vi "create_Karte.vi"() -> ()   [LabVIEW 2019]
uses:
  Karte.ctl
  Kreuzung.ctl
  Koordinate.ctl
  Strasse.ctl
  Verbindung.ctl
  Strassentyp.ctl
  Haus.ctl
  <vilib>/Utility/file.llb/Read Delimited Spreadsheet (string).vi
  <vilib>/Utility/xml.llb/Write to XML File(string).vi
panel:
  out "error out":errorcluster
  in  "OK Button":bool
  in  "Table Control":string[][](table)=[["", "", "", "", "", "", "", "s", "", "", "", "", "", "", "", "", "", "", "", "", "", "", "", "", ""], ["", "", "i", "", "", "", "", "", "", "", "", "", "", "", "", "", "", "", "", "", "", "", "", "", ""], ["", "i", "", "i", "", "", "", "", "", "", "i", "", "", "", "", "", "", "", "", "", "", "", "", "", ""], ["", "", "i", "", "i", "", "", "", "", "", "", "", "", "", "", "", "", "", "", "", "", "", "", "", ""], ["", "", "", "i", "", "", "", "", "", "", "", "", "", "", "", "", "", "", "", "", "", "", "", "", ""], ["", "", "", "", "", "", "s", "", "", "", "", "", "", "", "", "", "", "", "", "", "", "", "", "", ""], ["", "", "", "", "", "s", "", "s", "s", "", "", "", "", "", "", "", "", "", "", "", "", "", "", "", ""], ["s", "", "", "", "", "", "s", "", "", "", "", "", "", "", "", "", "", "", "", "", "", "", "", "", ""], ["", "", "", "", "", "", "s", "", "", "i", "", "", "", "", "", "", "", "", "s", "", "", "", "", "", ""], ["", "", "", "", "", "", "", "", "i", "", "i", "i", "", "", "", "", "", "", "", "", "", "", "", "", ""], ["", "", "i", "", "", "", "", "", "", "i", "", "", "i", "", "", "", "", "", "", "", "", "", "", "", ""], ["", "", "", "", "", "", "", "", "", "i", "", "", "i", "", "", "", "", "i", "", "", "", "", "", "", ""], ["", "", "", "", "", "", "", "", "", "", "i", "i", "", "i", "", "", "", "", "", "", "", "", "", "", ""], ["", "", "", "", "", "", "", "", "", "", "", "", "i", "", "i", "i", "", "", "", "", "", "", "", "", ""], ["", "", "", "i", "", "", "", "", "", "", "", "", "", "i", "", "", "", "", "", "", "", "", "", "", ""], ["", "", "", "", "", "", "", "", "", "", "", "", "", "i", "", "", "s", "", "", "", "", "", "", "s", ""], ["", "", "", "", "", "", "", "", "", "", "", "", "", "", "", "s", "", "", "", "", "", "", "", "", ""], ["", "", "", "", "", "", "", "", "", "", "", "i", "", "", "", "", "", "", "", "", "", "", "", "", ""], ["", "", "", "", "", "", "", "", "s", "", "", "", "", "", "", "", "", "", "", "", "", "", "", "", ""], ["", "", "", "", "", "", "", "", "", "", "", "", "", "", "", "", "", "", "", "", "a", "a", "", "", ""], ["", "", "", "", "", "", "", "", "", "", "", "", "", "", "", "", "", "", "", "a", "", "", "a", "", ""], ["", "", "", "", "", "", "", "", "", "", "", "", "", "", "", "", "", "", "", "a", "", "", "", "", ""], ["", "", "", "", "", "", "", "", "", "", "", "", "", "", "", "", "", "", "", "", "a", "", "", "a", ""], ["", "", "", "", "", "", "", "", "", "", "", "", "", "", "", "s", "", "", "", "", "", "", "a", "", "a"], ["", "", "", "", "", "", "", "", "", "", "", "", "", "", "", "", "", "", "", "", "", "", "", "a", ""]]
  in  "Nr Häuser":i32=20
  in  "Nr Kreuzungen":i32=25
  out "all rows":string[][](array[string])=[["Nr.", "X-DIM", "Y-DIM", "Typ", "", "", ""], ["A1", "100", "40", "Strasse", "", "", ""], ["A2", "180", "70", "Strasse", "", "", ""], ["A3", "210", "70", "Strasse", "", "", ""], ["A4", "300", "70", "Strasse", "", "", ""], ["A5", "320", "70", "Strasse", "", "", ""], ["A6", "40", "100", "Strasse", "", "", ""], ["A7", "90", "100", "Strasse", "", "", ""], ["A8", "100", "100", "Strasse", "", "", ""], ["A9", "90", "170", "Strasse", "", "", ""], ["A10", "180", "170", "Strasse", "", "", ""], ["A11", "210", "170", "Strasse", "", "", ""], ["A12", "180", "190", "Strasse", "", "", ""], ["A13", "210", "190", "Strasse", "", "", ""], ["A14", "270", "190", "Strasse", "", "", ""], ["A15", "300", "190", "Strasse", "", "", ""], ["A16", "270", "230", "Strasse", "", "", ""], ["A17", "340", "230", "Strasse", "", "", ""], ["A18", "180", "240", "Strasse", "", "", ""], ["A19", "90", "260", "Strasse", "", "", ""], ["A20", "60", "320", "Strasse", "", "", ""], ["A21", "160", "320", "Strasse", "", "", ""], ["A22", "60", "360", "Strasse", "", "", ""], ["A23", "160", "400", "Strasse", "", "", ""], ["A24", "270", "400", "Strasse", "", "", ""], ["A25", "340", "400", "Strasse", "", "", ""], ["B1", "160", "0", "Haus", "", "", ""], ["B2", "220", "0", "Haus", "", "", ""], ["B3", "220", "0", "Haus", "", "", ""], ["B4", "280", "0", "Haus", "", "", ""], ["B5", "280", "0", "Haus", "", "", ""], ["B6", "340", "0", "Haus", "", "", ""], ["B7", "20", "20", "Haus", "", "", ""], ["B8", "80", "20", "Haus", "", "", ""], ["B9", "190", "20", "Haus", "", "", ""], ["B10", "250", "20", "Haus", "", "", ""], ["B11", "310", "20", "Haus", "", "", ""], ["B12", "220", "40", "Haus", "", "", ""], ["B13", "280", "40", "Haus", "", "", ""], ["B14", "50", "40", "Haus", "", "", ""], ["B15", "120", "40", "Haus", "", "", ""], ["B16", "160", "40", "Haus", "", "", ""], ["B17", "220", "40", "Haus", "", "", ""], ["B18", "280", "40", "Haus", "", "", ""], ["B19", "340", "40", "Haus", "", "", ""], ["B20", "340", "40", "Haus", "", "", ""], ["B21", "160", "40", "Haus", "", "", ""], ["B22", "380", "40", "Haus", "", "", ""], ["B23", "20", "60", "Haus", "", "", ""], ["B24", "80", "60", "Haus", "", "", ""], ["B25", "140", "70", "Haus", "", "", ""], ["B26", "360", "70", "Haus", "", "", ""], ["B27", "160", "100", "Haus", "", "", ""], ["B28", "380", "100", "Haus", "", "", ""], ["B29", "120", "100", "Haus", "", "", ""], ["B30", "120", "100", "Haus", "", "", ""], ["B31", "180", "100", "Haus", "", "", ""], ["B32", "240", "100", "Haus", "", "", ""], ["B33", "340", "100", "Haus", "", "", ""], ["B34", "380", "100", "Haus", "", "", ""], ["B35", "280", "100", "Haus", "", "", ""], ["B36", "320", "100", "Haus", "", "", ""], ["B37", "20", "120", "Haus", "", "", ""], ["B38", "60", "120", "Haus", "", "", ""], ["B39", "150", "120", "Haus", "", "", ""], ["B40", "350", "120", "Haus", "", "", ""], ["B41", "260", "130", "Haus", "", "", ""], ["B42", "180", "140", "Haus", "", "", ""], ["B43", "120", "140", "Haus", "", "", ""], ["B44", "320", "140", "Haus", "", "", ""], ["B45", "320", "140", "Haus", "", "", ""], ["B46", "380", "140", "Haus", "", "", ""], ["B47", "360", "140", "Haus", "", "", ""], ["B48", "40", "150", "Haus", "", "", ""], ["B49", "280", "160", "Haus", "", "", ""], ["B50", "240", "160", "Haus", "", "", ""], ["B51", "340", "170", "Haus", "", "", ""], ["B52", "20", "180", "Haus", "", "", ""], ["B53", "60", "180", "Haus", "", "", ""], ["B54", "45", "180", "Haus", "", "", ""], ["B55", "5", "180", "Haus", "", "", ""], ["B56", "360", "200", "Haus", "", "", ""], ["B57", "160", "200", "Haus", "", "", ""], ["B58", "320", "200", "Haus", "", "", ""], ["B59", "120", "200", "Haus", "", "", ""], ["B60", "25", "210", "Haus", "", "", ""], ["B61", "200", "220", "Haus", "", "", ""], ["B62", "240", "220", "Haus", "", "", ""], ["B63", "140", "230", "Haus", "", "", ""], ["B64", "5", "240", "Haus", "", "", ""], ["B65", "0", "240", "Haus", "", "", ""], ["B66", "45", "240", "Haus", "", "", ""], ["B67", "60", "240", "Haus", "", "", ""], ["B68", "220", "250", "Haus", "", "", ""], ["B69", "120", "260", "Haus", "", "", ""], ["B70", "30", "260", "Haus", "", "", ""], ["B71", "130", "260", "Haus", "", "", ""], ["B72", "160", "260", "Haus", "", "", ""], ["B73", "190", "260", "Haus", "", "", ""], ["B74", "60", "280", "Haus", "", "", ""], ["B75", "200", "280", "Haus", "", "", ""], ["B76", "240", "280", "Haus", "", "", ""], ["B77", "0", "280", "Haus", "", "", ""], ["B78", "160", "280", "Haus", "", "", ""], ["B79", "300", "280", "Haus", "", "", ""], ["B80", "360", "280", "Haus", "", "", ""], ["B81", "240", "290", "Haus", "", "", ""], ["B82", "200", "290", "Haus", "", "", ""], ["B83", "130", "300", "Haus", "", "", ""], ["B84", "190", "300", "Haus", "", "", ""], ["B85", "330", "300", "Haus", "", "", ""], ["B86", "220", "320", "Haus", "", "", ""], ["B87", "300", "320", "Haus", "", "", ""], ["B88", "360", "320", "Haus", "", "", ""], ["B89", "300", "320", "Haus", "", "", ""], ["B90", "360", "320", "Haus", "", "", ""], ["B91", "330", "340", "Haus", "", "", ""], ["B92", "200", "350", "Haus", "", "", ""], ["B93", "240", "350", "Haus", "", "", ""], ["B94", "300", "360", "Haus", "", "", ""], ["B95", "360", "360", "Haus", "", "", ""], ["B96", "30", "400", "Haus", "", "", ""], ["B97", "90", "400", "Haus", "", "", ""], ["B98", "60", "420", "Haus", "", "", ""], ["B99", "30", "440", "Haus", "", "", ""], ["B100", "90", "440", "Haus", "", "", ""], ["C1", "250", "40", "Haustüre", "", "", ""], ["C2", "310", "40", "Haustüre", "", "", ""], ["C3", "50", "60", "Haustüre", "", "", ""], ["C4", "120", "70", "Haustüre", "", "", ""], ["C5", "340", "70", "Haustüre", "", "", ""], ["C6", "40", "120", "Haustüre", "", "", ""], ["C7", "180", "120", "Haustüre", "", "", ""], ["C8", "320", "120", "Haustüre", "", "", ""], ["C9", "240", "130", "Haustüre", "", "", ""], ["C10", "320", "170", "Haustüre", "", "", ""], ["C11", "45", "210", "Haustüre", "", "", ""], ["C12", "220", "220", "Haustüre", "", "", ""], ["C13", "160", "230", "Haustüre", "", "", ""], ["C14", "60", "260", "Haustüre", "", "", ""], ["C15", "330", "280", "Haustüre", "", "", ""], ["C16", "160", "300", "Haustüre", "", "", ""], ["C17", "240", "320", "Haustüre", "", "", ""], ["C18", "330", "360", "Haustüre", "", "", ""], ["C19", "60", "400", "Haustüre", "", "", ""], ["D1", "190", "40", "Poststelle", "", "", ""]]
  in  "Path":path=path "C:/Users/juerg.keller1/Documents/FHNW/STUDPROJ/2019_2020/APAS/labview/Parcelcity_Training_V2.3.csv"
  out "Karte":T1={"Kreuzungen"=[{"Name"="A1", "Identifikation"=0, "Koord"={"x"=100.0, "y"=100.0}, "Anzahl Abgänge"=1}, {"Name"="A2", "Identifikation"=1, "Koord"={"x"=180.0, "y"=180.0}, "Anzahl Abgänge"=1}, {"Name"="A3", "Identifikation"=2, "Koord"={"x"=210.0, "y"=210.0}, "Anzahl Abgänge"=3}, {"Name"="A4", "Identifikation"=3, "Koord"={"x"=300.0, "y"=300.0}, "Anzahl Abgänge"=3}, {"Name"="A5", "Identifikation"=4, "Koord"={"x"=320.0, "y"=320.0}, "Anzahl Abgänge"=1}, {"Name"="A6", "Identifikation"=5, "Koord"={"x"=40.0, "y"=40.0}, "Anzahl Abgänge"=1}, {"Name"="A7", "Identifikation"=6, "Koord"={"x"=90.0, "y"=90.0}, "Anzahl Abgänge"=3}, {"Name"="A8", "Identifikation"=7, "Koord"={"x"=100.0, "y"=100.0}, "Anzahl Abgänge"=2}, {"Name"="A9", "Identifikation"=8, "Koord"={"x"=90.0, "y"=90.0}, "Anzahl Abgänge"=2}, {"Name"="A10", "Identifikation"=9, "Koord"={"x"=180.0, "y"=180.0}, "Anzahl Abgänge"=4}, {"Name"="A11", "Identifikation"=10, "Koord"={"x"=210.0, "y"=210.0}, "Anzahl Abgänge"=3}, {"Name"="A12", "Identifikation"=11, "Koord"={"x"=180.0, "y"=180.0}, "Anzahl Abgänge"=3}, {"Name"="A13", "Identifikation"=12, "Koord"={"x"=210.0, "y"=210.0}, "Anzahl Abgänge"=3}, {"Name"="A14", "Identifikation"=13, "Koord"={"x"=270.0, "y"=270.0}, "Anzahl Abgänge"=3}, {"Name"="A15", "Identifikation"=14, "Koord"={"x"=300.0, "y"=300.0}, "Anzahl Abgänge"=1}, {"Name"="A16", "Identifikation"=15, "Koord"={"x"=270.0, "y"=270.0}, "Anzahl Abgänge"=3}, {"Name"="A17", "Identifikation"=16, "Koord"={"x"=340.0, "y"=340.0}, "Anzahl Abgänge"=1}, {"Name"="A18", "Identifikation"=17, "Koord"={"x"=180.0, "y"=180.0}, "Anzahl Abgänge"=1}, {"Name"="A19", "Identifikation"=18, "Koord"={"x"=90.0, "y"=90.0}, "Anzahl Abgänge"=1}, {"Name"="A20", "Identifikation"=19, "Koord"={"x"=60.0, "y"=60.0}, "Anzahl Abgänge"=2}, {"Name"="A21", "Identifikation"=20, "Koord"={"x"=160.0, "y"=160.0}, "Anzahl Abgänge"=2}, {"Name"="A22", "Identifikation"=21, "Koord"={"x"=60.0, "y"=60.0}, "Anzahl Abgänge"=1}, {"Name"="A23", "Identifikation"=22, "Koord"={"x"=160.0, "y"=160.0}, "Anzahl Abgänge"=2}, {"Name"="A24", "Identifikation"=23, "Koord"={"x"=270.0, "y"=270.0}, "Anzahl Abgänge"=3}, {"Name"="A25", "Identifikation"=24, "Koord"={"x"=340.0, "y"=340.0}, "Anzahl Abgänge"=1}], "Strassen"=[{"Name"="A 1 8", "Identifikation"=0, "Verbindungen"=[{"Start_Kr"=0, "Ziel_Kr"=7}], "Breite"=40, "Strassen_Typ"=enum."Stadt"}, {"Name"="A 2 3", "Identifikation"=1, "Verbindungen"=[{"Start_Kr"=1, "Ziel_Kr"=2}], "Breite"=60, "Strassen_Typ"=enum."Innenstadt"}, {"Name"="A 2 3", "Identifikation"=1, "Verbindungen"=[{"Start_Kr"=1, "Ziel_Kr"=2}, {"Start_Kr"=2, "Ziel_Kr"=1}], "Breite"=60, "Strassen_Typ"=enum."Innenstadt"}, {"Name"="A 3 4", "Identifikation"=3, "Verbindungen"=[{"Start_Kr"=2, "Ziel_Kr"=3}], "Breite"=60, "Strassen_Typ"=enum."Innenstadt"}, {"Name"="A 311", "Identifikation"=4, "Verbindungen"=[{"Start_Kr"=2, "Ziel_Kr"=10}], "Breite"=60, "Strassen_Typ"=enum."Innenstadt"}, {"Name"="A 3 4", "Identifikation"=3, "Verbindungen"=[{"Start_Kr"=2, "Ziel_Kr"=3}, {"Start_Kr"=3, "Ziel_Kr"=2}], "Breite"=60, "Strassen_Typ"=enum."Innenstadt"}, {"Name"="A 4 5", "Identifikation"=6, "Verbindungen"=[{"Start_Kr"=3, "Ziel_Kr"=4}], "Breite"=60, "Strassen_Typ"=enum."Innenstadt"}, {"Name"="A 4 5", "Identifikation"=6, "Verbindungen"=[{"Start_Kr"=3, "Ziel_Kr"=4}, {"Start_Kr"=4, "Ziel_Kr"=3}], "Breite"=60, "Strassen_Typ"=enum."Innenstadt"}, {"Name"="A 6 7", "Identifikation"=8, "Verbindungen"=[{"Start_Kr"=5, "Ziel_Kr"=6}], "Breite"=40, "Strassen_Typ"=enum."Stadt"}, {"Name"="A 6 7", "Identifikation"=8, "Verbindungen"=[{"Start_Kr"=5, "Ziel_Kr"=6}, {"Start_Kr"=6, "Ziel_Kr"=5}], "Breite"=40, "Strassen_Typ"=enum."Stadt"}, {"Name"="A 7 8", "Identifikation"=10, "Verbindungen"=[{"Start_Kr"=6, "Ziel_Kr"=7}], "Breite"=40, "Strassen_Typ"=enum."Stadt"}, {"Name"="A 7 9", "Identifikation"=11, "Verbindungen"=[{"Start_Kr"=6, "Ziel_Kr"=8}], "Breite"=40, "Strassen_Typ"=enum."Stadt"}, {"Name"="A 1 8", "Identifikation"=0, "Verbindungen"=[{"Start_Kr"=0, "Ziel_Kr"=7}, {"Start_Kr"=7, "Ziel_Kr"=0}], "Breite"=40, "Strassen_Typ"=enum."Stadt"}, {"Name"="A 7 8", "Identifikation"=10, "Verbindungen"=[{"Start_Kr"=6, "Ziel_Kr"=7}, {"Start_Kr"=7, "Ziel_Kr"=6}], "Breite"=40, "Strassen_Typ"=enum."Stadt"}, {"Name"="A 7 9", "Identifikation"=11, "Verbindungen"=[{"Start_Kr"=6, "Ziel_Kr"=8}, {"Start_Kr"=8, "Ziel_Kr"=6}], "Breite"=40, "Strassen_Typ"=enum."Stadt"}, {"Name"="A 910", "Identifikation"=15, "Verbindungen"=[{"Start_Kr"=8, "Ziel_Kr"=9}], "Breite"=40, "Strassen_Typ"=enum."Innenstadt"}, {"Name"="A 919", "Identifikation"=16, "Verbindungen"=[{"Start_Kr"=8, "Ziel_Kr"=18}], "Breite"=40, "Strassen_Typ"=enum."Stadt"}, {"Name"="A 910", "Identifikation"=15, "Verbindungen"=[{"Start_Kr"=8, "Ziel_Kr"=9}, {"Start_Kr"=9, "Ziel_Kr"=8}], "Breite"=40, "Strassen_Typ"=enum."Innenstadt"}, {"Name"="A1011", "Identifikation"=18, "Verbindungen"=[{"Start_Kr"=9, "Ziel_Kr"=10}], "Breite"=40, "Strassen_Typ"=enum."Innenstadt"}, {"Name"="A1012", "Identifikation"=19, "Verbindungen"=[{"Start_Kr"=9, "Ziel_Kr"=11}], "Breite"=40, "Strassen_Typ"=enum."Innenstadt"}, {"Name"="A 311", "Identifikation"=4, "Verbindungen"=[{"Start_Kr"=2, "Ziel_Kr"=10}, {"Start_Kr"=10, "Ziel_Kr"=2}], "Breite"=60, "Strassen_Typ"=enum."Innenstadt"}, {"Name"="A1011", "Identifikation"=18, "Verbindungen"=[{"Start_Kr"=9, "Ziel_Kr"=10}, {"Start_Kr"=10, "Ziel_Kr"=9}], "Breite"=40, "Strassen_Typ"=enum."Innenstadt"}, {"Name"="A1113", "Identifikation"=22, "Verbindungen"=[{"Start_Kr"=10, "Ziel_Kr"=12}], "Breite"=40, "Strassen_Typ"=enum."Innenstadt"}, {"Name"="A1012", "Identifikation"=19, "Verbindungen"=[{"Start_Kr"=9, "Ziel_Kr"=11}, {"Start_Kr"=11, "Ziel_Kr"=9}], "Breite"=40, "Strassen_Typ"=enum."Innenstadt"}, {"Name"="A1213", "Identifikation"=24, "Verbindungen"=[{"Start_Kr"=11, "Ziel_Kr"=12}], "Breite"=40, "Strassen_Typ"=enum."Innenstadt"}, {"Name"="A1218", "Identifikation"=25, "Verbindungen"=[{"Start_Kr"=11, "Ziel_Kr"=17}], "Breite"=40, "Strassen_Typ"=enum."Innenstadt"}, {"Name"="A1113", "Identifikation"=22, "Verbindungen"=[{"Start_Kr"=10, "Ziel_Kr"=12}, {"Start_Kr"=12, "Ziel_Kr"=10}], "Breite"=40, "Strassen_Typ"=enum."Innenstadt"}, {"Name"="A1213", "Identifikation"=24, "Verbindungen"=[{"Start_Kr"=11, "Ziel_Kr"=12}, {"Start_Kr"=12, "Ziel_Kr"=11}], "Breite"=40, "Strassen_Typ"=enum."Innenstadt"}, {"Name"="A1314", "Identifikation"=28, "Verbindungen"=[{"Start_Kr"=12, "Ziel_Kr"=13}], "Breite"=40, "Strassen_Typ"=enum."Innenstadt"}, {"Name"="A1314", "Identifikation"=28, "Verbindungen"=[{"Start_Kr"=12, "Ziel_Kr"=13}, {"Start_Kr"=13, "Ziel_Kr"=12}], "Breite"=40, "Strassen_Typ"=enum."Innenstadt"}, {"Name"="A1415", "Identifikation"=30, "Verbindungen"=[{"Start_Kr"=13, "Ziel_Kr"=14}], "Breite"=40, "Strassen_Typ"=enum."Innenstadt"}, {"Name"="A1416", "Identifikation"=31, "Verbindungen"=[{"Start_Kr"=13, "Ziel_Kr"=15}], "Breite"=40, "Strassen_Typ"=enum."Innenstadt"}, {"Name"="A 415", "Identifikation"=32, "Verbindungen"=[{"Start_Kr"=14, "Ziel_Kr"=3}], "Breite"=40, "Strassen_Typ"=enum."Innenstadt"}, {"Name"="A1415", "Identifikation"=30, "Verbindungen"=[{"Start_Kr"=13, "Ziel_Kr"=14}, {"Start_Kr"=14, "Ziel_Kr"=13}], "Breite"=40, "Strassen_Typ"=enum."Innenstadt"}, {"Name"="A1416", "Identifikation"=31, "Verbindungen"=[{"Start_Kr"=13, "Ziel_Kr"=15}, {"Start_Kr"=15, "Ziel_Kr"=13}], "Breite"=40, "Strassen_Typ"=enum."Innenstadt"}, {"Name"="A1617", "Identifikation"=35, "Verbindungen"=[{"Start_Kr"=15, "Ziel_Kr"=16}], "Breite"=40, "Strassen_Typ"=enum."Stadt"}, {"Name"="A1624", "Identifikation"=36, "Verbindungen"=[{"Start_Kr"=15, "Ziel_Kr"=23}], "Breite"=40, "Strassen_Typ"=enum."Stadt"}, {"Name"="A1617", "Identifikation"=35, "Verbindungen"=[{"Start_Kr"=15, "Ziel_Kr"=16}, {"Start_Kr"=16, "Ziel_Kr"=15}], "Breite"=40, "Strassen_Typ"=enum."Stadt"}, {"Name"="A1218", "Identifikation"=25, "Verbindungen"=[{"Start_Kr"=11, "Ziel_Kr"=17}, {"Start_Kr"=17, "Ziel_Kr"=11}], "Breite"=40, "Strassen_Typ"=enum."Innenstadt"}, {"Name"="A1019", "Identifikation"=39, "Verbindungen"=[{"Start_Kr"=18, "Ziel_Kr"=9}], "Breite"=40, "Strassen_Typ"=enum."Stadt"}, {"Name"="A2021", "Identifikation"=40, "Verbindungen"=[{"Start_Kr"=19, "Ziel_Kr"=20}], "Breite"=40, "Strassen_Typ"=enum."Land"}, {"Name"="A2022", "Identifikation"=41, "Verbindungen"=[{"Start_Kr"=19, "Ziel_Kr"=21}], "Breite"=40, "Strassen_Typ"=enum."Land"}, {"Name"="A2021", "Identifikation"=40, "Verbindungen"=[{"Start_Kr"=19, "Ziel_Kr"=20}, {"Start_Kr"=20, "Ziel_Kr"=19}], "Breite"=40, "Strassen_Typ"=enum."Land"}, {"Name"="A2123", "Identifikation"=43, "Verbindungen"=[{"Start_Kr"=20, "Ziel_Kr"=22}], "Breite"=40, "Strassen_Typ"=enum."Land"}, {"Name"="A2022", "Identifikation"=41, "Verbindungen"=[{"Start_Kr"=19, "Ziel_Kr"=21}, {"Start_Kr"=21, "Ziel_Kr"=19}], "Breite"=40, "Strassen_Typ"=enum."Land"}, {"Name"="A2123", "Identifikation"=43, "Verbindungen"=[{"Start_Kr"=20, "Ziel_Kr"=22}, {"Start_Kr"=22, "Ziel_Kr"=20}], "Breite"=40, "Strassen_Typ"=enum."Land"}, {"Name"="A2324", "Identifikation"=46, "Verbindungen"=[{"Start_Kr"=22, "Ziel_Kr"=23}], "Breite"=40, "Strassen_Typ"=enum."Land"}, {"Name"="A1624", "Identifikation"=36, "Verbindungen"=[{"Start_Kr"=15, "Ziel_Kr"=23}, {"Start_Kr"=23, "Ziel_Kr"=15}], "Breite"=40, "Strassen_Typ"=enum."Stadt"}, {"Name"="A2324", "Identifikation"=46, "Verbindungen"=[{"Start_Kr"=22, "Ziel_Kr"=23}, {"Start_Kr"=23, "Ziel_Kr"=22}], "Breite"=40, "Strassen_Typ"=enum."Land"}, {"Name"="A2425", "Identifikation"=49, "Verbindungen"=[{"Start_Kr"=23, "Ziel_Kr"=24}], "Breite"=40, "Strassen_Typ"=enum."Land"}, {"Name"="A2425", "Identifikation"=49, "Verbindungen"=[{"Start_Kr"=23, "Ziel_Kr"=24}, {"Start_Kr"=24, "Ziel_Kr"=23}], "Breite"=40, "Strassen_Typ"=enum."Land"}], "Häuser"=[{"Name"="Haus1", "Hausnummer"=0, "Polygon"=[{"x"=220.0, "y"=40.0}, {"x"=280.0, "y"=40.0}, {"x"=280.0, "y"=0.0}, {"x"=220.0, "y"=0.0}, {"x"=250.0, "y"=20.0}], "Strassennummer"=0, "Türe"={"x"=250.0, "y"=40.0}}, {"Name"="Haus2", "Hausnummer"=1, "Polygon"=[{"x"=280.0, "y"=40.0}, {"x"=340.0, "y"=40.0}, {"x"=340.0, "y"=0.0}, {"x"=280.0, "y"=0.0}, {"x"=310.0, "y"=20.0}], "Strassennummer"=0, "Türe"={"x"=310.0, "y"=40.0}}, {"Name"="Haus3", "Hausnummer"=2, "Polygon"=[{"x"=20.0, "y"=60.0}, {"x"=80.0, "y"=60.0}, {"x"=80.0, "y"=20.0}, {"x"=20.0, "y"=20.0}, {"x"=50.0, "y"=40.0}], "Strassennummer"=0, "Türe"={"x"=50.0, "y"=60.0}}, {"Name"="Haus4", "Hausnummer"=3, "Polygon"=[{"x"=120.0, "y"=40.0}, {"x"=120.0, "y"=100.0}, {"x"=160.0, "y"=100.0}, {"x"=160.0, "y"=40.0}, {"x"=140.0, "y"=70.0}], "Strassennummer"=0, "Türe"={"x"=120.0, "y"=70.0}}, {"Name"="Haus5", "Hausnummer"=4, "Polygon"=[{"x"=340.0, "y"=40.0}, {"x"=340.0, "y"=100.0}, {"x"=380.0, "y"=100.0}, {"x"=380.0, "y"=40.0}, {"x"=360.0, "y"=70.0}], "Strassennummer"=0, "Türe"={"x"=340.0, "y"=70.0}}, {"Name"="Haus6", "Hausnummer"=5, "Polygon"=[{"x"=20.0, "y"=120.0}, {"x"=20.0, "y"=180.0}, {"x"=60.0, "y"=180.0}, {"x"=60.0, "y"=120.0}, {"x"=40.0, "y"=150.0}], "Strassennummer"=0, "Türe"={"x"=40.0, "y"=120.0}}, {"Name"="Haus7", "Hausnummer"=6, "Polygon"=[{"x"=180.0, "y"=100.0}, {"x"=120.0, "y"=100.0}, {"x"=120.0, "y"=140.0}, {"x"=180.0, "y"=140.0}, {"x"=150.0, "y"=120.0}], "Strassennummer"=0, "Türe"={"x"=180.0, "y"=120.0}}, {"Name"="Haus8", "Hausnummer"=7, "Polygon"=[{"x"=320.0, "y"=140.0}, {"x"=380.0, "y"=140.0}, {"x"=380.0, "y"=100.0}, {"x"=320.0, "y"=100.0}, {"x"=350.0, "y"=120.0}], "Strassennummer"=0, "Türe"={"x"=320.0, "y"=120.0}}, {"Name"="Haus9", "Hausnummer"=8, "Polygon"=[{"x"=240.0, "y"=100.0}, {"x"=240.0, "y"=160.0}, {"x"=280.0, "y"=160.0}, {"x"=280.0, "y"=100.0}, {"x"=260.0, "y"=130.0}], "Strassennummer"=0, "Türe"={"x"=240.0, "y"=130.0}}, {"Name"="Haus10", "Hausnummer"=9, "Polygon"=[{"x"=320.0, "y"=140.0}, {"x"=320.0, "y"=200.0}, {"x"=360.0, "y"=200.0}, {"x"=360.0, "y"=140.0}, {"x"=340.0, "y"=170.0}], "Strassennummer"=0, "Türe"={"x"=320.0, "y"=170.0}}, {"Name"="Haus11", "Hausnummer"=10, "Polygon"=[{"x"=45.0, "y"=240.0}, {"x"=45.0, "y"=180.0}, {"x"=5.0, "y"=180.0}, {"x"=5.0, "y"=240.0}, {"x"=25.0, "y"=210.0}], "Strassennummer"=0, "Türe"={"x"=45.0, "y"=210.0}}, {"Name"="Haus12", "Hausnummer"=11, "Polygon"=[{"x"=200.0, "y"=220.0}, {"x"=200.0, "y"=280.0}, {"x"=240.0, "y"=280.0}, {"x"=240.0, "y"=220.0}, {"x"=220.0, "y"=250.0}], "Strassennummer"=0, "Türe"={"x"=220.0, "y"=220.0}}, {"Name"="Haus13", "Hausnummer"=12, "Polygon"=[{"x"=160.0, "y"=260.0}, {"x"=160.0, "y"=200.0}, {"x"=120.0, "y"=200.0}, {"x"=120.0, "y"=260.0}, {"x"=140.0, "y"=230.0}], "Strassennummer"=0, "Türe"={"x"=160.0, "y"=230.0}}, {"Name"="Haus14", "Hausnummer"=13, "Polygon"=[{"x"=60.0, "y"=240.0}, {"x"=0.0, "y"=240.0}, {"x"=0.0, "y"=280.0}, {"x"=60.0, "y"=280.0}, {"x"=30.0, "y"=260.0}], "Strassennummer"=0, "Türe"={"x"=60.0, "y"=260.0}}, {"Name"="Haus15", "Hausnummer"=14, "Polygon"=[{"x"=360.0, "y"=280.0}, {"x"=300.0, "y"=280.0}, {"x"=300.0, "y"=320.0}, {"x"=360.0, "y"=320.0}, {"x"=330.0, "y"=300.0}], "Strassennummer"=0, "Türe"={"x"=330.0, "y"=280.0}}, {"Name"="Haus16", "Hausnummer"=15, "Polygon"=[{"x"=130.0, "y"=300.0}, {"x"=190.0, "y"=300.0}, {"x"=190.0, "y"=260.0}, {"x"=130.0, "y"=260.0}, {"x"=160.0, "y"=280.0}], "Strassennummer"=0, "Türe"={"x"=160.0, "y"=300.0}}, {"Name"="Haus17", "Hausnummer"=16, "Polygon"=[{"x"=240.0, "y"=350.0}, {"x"=240.0, "y"=290.0}, {"x"=200.0, "y"=290.0}, {"x"=200.0, "y"=350.0}, {"x"=220.0, "y"=320.0}], "Strassennummer"=0, "Türe"={"x"=240.0, "y"=320.0}}, {"Name"="Haus18", "Hausnummer"=17, "Polygon"=[{"x"=300.0, "y"=360.0}, {"x"=360.0, "y"=360.0}, {"x"=360.0, "y"=320.0}, {"x"=300.0, "y"=320.0}, {"x"=330.0, "y"=340.0}], "Strassennummer"=0, "Türe"={"x"=330.0, "y"=360.0}}, {"Name"="Haus19", "Hausnummer"=18, "Polygon"=[{"x"=90.0, "y"=400.0}, {"x"=30.0, "y"=400.0}, {"x"=30.0, "y"=440.0}, {"x"=90.0, "y"=440.0}, {"x"=60.0, "y"=420.0}], "Strassennummer"=0, "Türe"={"x"=60.0, "y"=400.0}}, {"Name"="Poststelle", "Hausnummer"=19, "Polygon"=[{"x"=160.0, "y"=40.0}, {"x"=220.0, "y"=40.0}, {"x"=220.0, "y"=0.0}, {"x"=160.0, "y"=0.0}, {"x"=190.0, "y"=20.0}], "Strassennummer"=0, "Türe"={"x"=190.0, "y"=40.0}}]}
  # "i: Innenstadt\ns: Stadt\na: aussen"
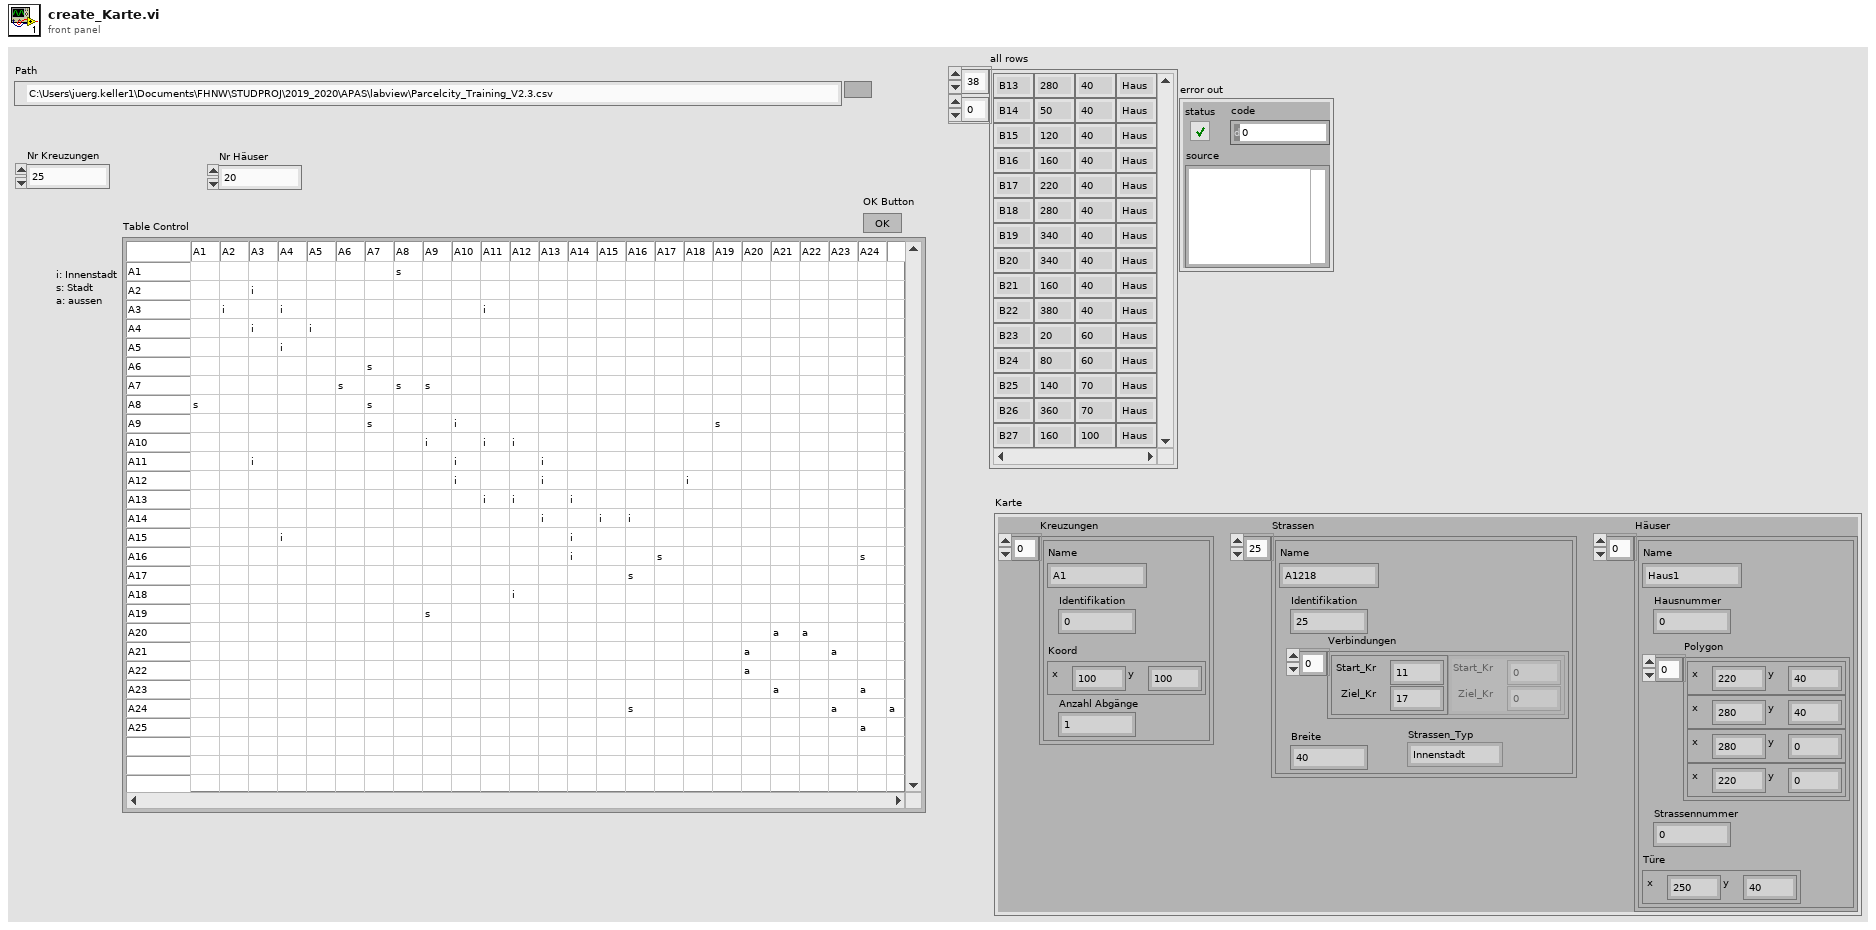
[diagram p1: front panel]
types:
  T1 = typedef "Karte.ctl" = cluster{"Kreuzungen":T2[], "Strassen":T4[], "Häuser":T7[]}
  T2 = typedef "Kreuzung.ctl" = cluster{"Name":string, "Identifikation":u8, "Koord":T3, "Anzahl Abgänge":u8}
  T3 = typedef "Koordinate.ctl" = cluster{"x":dbl, "y":dbl}
  T4 = typedef "Strasse.ctl" = cluster{"Name":string, "Identifikation":u8, "Verbindungen":T5[], "Breite":u8, "Strassen_Typ":T6}
  T5 = typedef "Verbindung.ctl" = cluster{"Start_Kr":u16, "Ziel_Kr":u16}
  T6 = typedef "Strassentyp.ctl" = enum16{"Innenstadt", "Stadt", "Land"}
  T7 = typedef "Haus.ctl" = cluster{"Name":string, "Hausnummer":u8, "Polygon":T3[], "Strassennummer":u8, "Türe":T3}
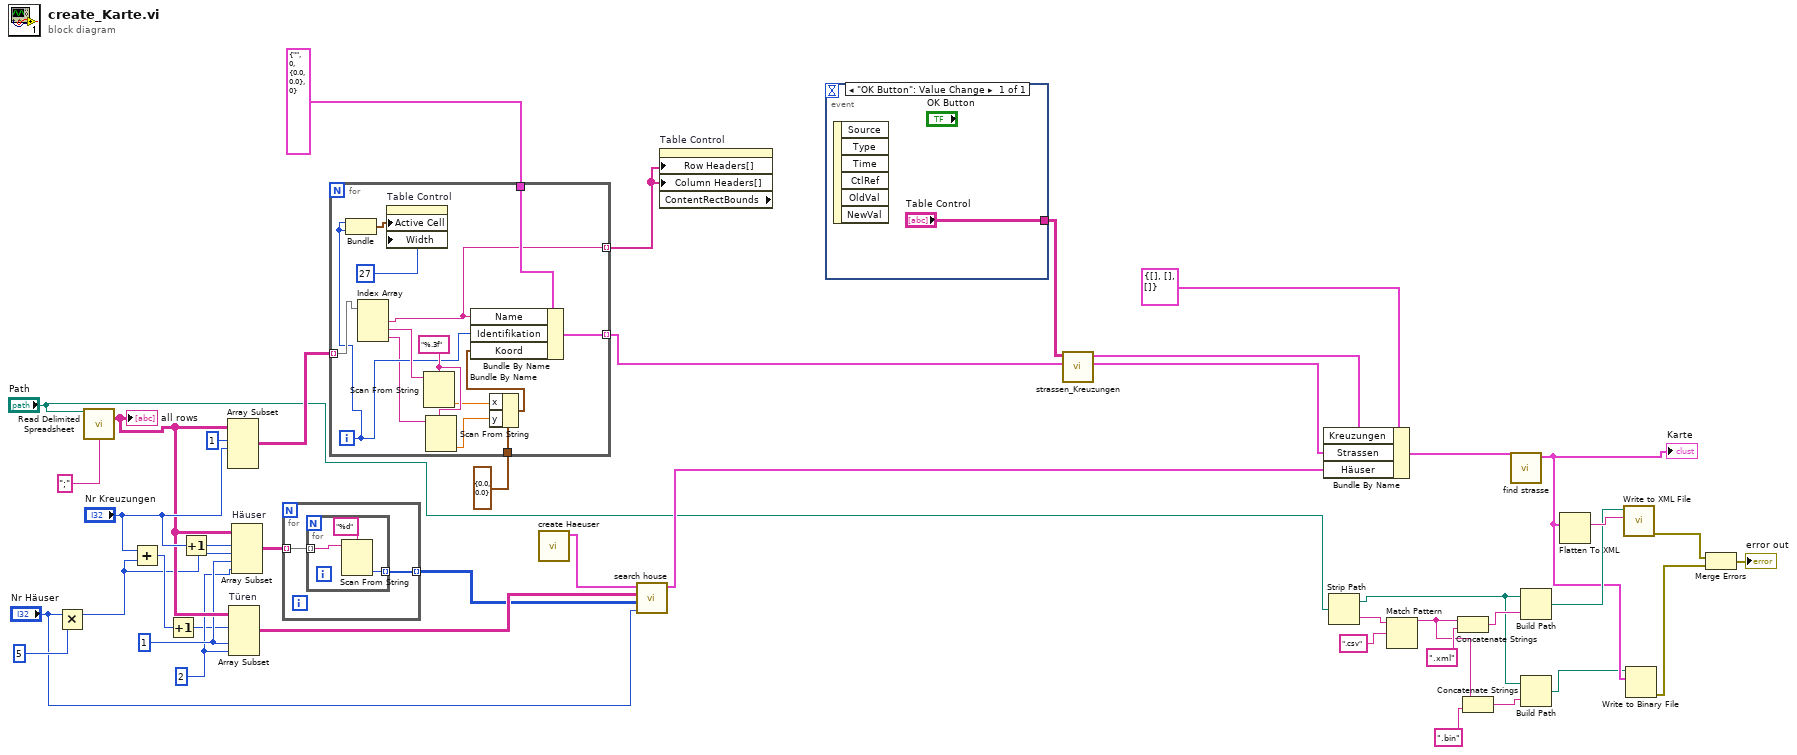
[diagram p0: block diagram]
diagram:
  w21 = 2 ("length")
  w22 = 1 ("index")
  n1 = Multiply(x="Nr Häuser", y=5) -> (x*y=w30:i32)
  n2 = call-poly <vilib>:"Read Delimited Spreadsheet.vi"("file path (dialog if empty)"="Path", "delimiter (\\t)"=";" ("delimiter (\\t)")) -> ("all rows"=w33:string[][])  [unwired: 8 in, 5 out]
  "all rows" <- w33
  n3 = Add(x="Nr Kreuzungen", y=w30) -> (x+y=w35:i32)
  n4 = Increment(x=w35) -> (x+1=w19:i32)
  n5 = Increment(x="Nr Kreuzungen") -> (x+1=w20:i32)
  n6 = Array Subset(array=w33, index (row)=1 ("index"), length (row)="Nr Kreuzungen") -> (w41:string[][])  [unwired: 2 in]
  n7 = Array Subset "Türen"(array=w33, index (row)=w19, index (col)=w22, length (col)=w21) -> (w31:string[][])  [unwired: 1 in]
  n8 = Array Subset "Häuser"(array=w33, index (row)=w20, length (row)=w30, index (col)=w22, length (col)=w21) -> (w32:string[][])
  n9 = for {
    tunnel: w32 -> [w45] mode=indexing
    tunnel: [w44] -> w28 mode=indexing
    n10 = for {
      tunnel: w45 -> [w48] mode=indexing
      tunnel: [w46] -> w44 mode=indexing
      n11 = Scan From String(format string="%d", input string=w48) -> (output 1=w46:i32)  [unwired: 3 in, 3 out]
    }
  }
  n12 = for {
    tunnel: w41 -> [w60] mode=indexing
    tunnel: T2 {"Name"="", "Identifikation"=0, "Koord"={"x"=0.0, "y"=0.0}, "Anzahl Abgänge"=0} ("Kreuzung") -> [w62]
    tunnel: T3 {"x"=0.0, "y"=0.0} ("Koord") -> [w61]
    tunnel: [w54] -> w36 mode=indexing
    tunnel: [w53] -> w38 mode=indexing
    i -> [w51]
    w58 = "%.3f" ("format string")
    n13 = Bundle(w51, w51) -> (w52:cluster{i32, i32})  [unwired: 1 in]
    n14 = Index Array(array=w60) -> (element #1=w53:string, element #2=w59:string, element #3=w49:string)  [unwired: 3 in]
    n15 = property on="Table Control" class="Tbl (strict)"("Active Cell"=w52, "Width"=u32 27 ("Active Cell:Cell Size:Width")) -> ()  [unwired: 2 in, 2 out]
    n16 = Scan From String(format string=w58, input string=w59) -> (output 1=w56:dbl)  [unwired: 3 in, 3 out]
    n17 = Scan From String(format string=w58, input string=w49) -> (output 1=w57:dbl)  [unwired: 3 in, 3 out]
    n18 = Bundle By Name(cluster=w61, "x"=w56, "y"=w57) -> (w55:T3)
    n19 = Bundle By Name(cluster=w62, "Name"=w53, "Identifikation"=w51, "Koord"=w55) -> (w54:T2)
  }
  n20 = call "create Haeuser.vi"() -> ("Häuser"=w27:cluster{i32[][]}[])  [unwired: 11 in]
  n21 = call "search house.vi"("Nr Türen"="Nr Häuser", "Häuser koord"=w28, "Türen"=w31, "Häuserlagen"=w27) -> ("Häuser"=w17:T7[])  [unwired: 7 in]
  n22 = property on="Table Control" class="Tbl (strict)" props=["Row Headers[]", "Column Headers[]", "ContentRectBounds"]("Row Headers[]"=w38, "Column Headers[]"=w38) -> ()  [unwired: 2 in, 3 out]
  n23 = event shown="[0] \"OK Button\": Value Change" {
    selector: _ -> [_]
    dyn-events: _ -> [_]
    timeout: _ -> [_]
    tunnel: ["Table Control"] -> w37
    event "OK Button": Value Change {
      n24 = event-data() -> ()  [unwired: 1 in, 6 out]
    }
  }
  n25 = call "strassen_Kreuzungen.vi"("Kreuzungen in"=w36, "Table Control"=w37) -> ("Strassen"=w24:T4[], "Kreuzungen out"=w23:T2[])  [unwired: 8 in]
  n26 = Bundle By Name(cluster=T1 {"Kreuzungen"=[], "Strassen"=[], "Häuser"=[]} ("Karte"), "Kreuzungen"=w23, "Strassen"=w24, "Häuser"=w17) -> (w25:T1)
  n27 = Strip Path(path="Path") -> (stripped path=w1:path, name=w15:string)
  n28 = Match Pattern(string=w15, regular expression=".csv") -> (before substring=w9:string)  [unwired: 1 in, 3 out]
  n29 = Concatenate Strings(w9, ".xml" ("string")) -> (w12:string)
  n30 = Concatenate Strings(w9, ".bin" ("string")) -> (w7:string)
  n31 = call "find strasse.vi"("Karte in"=w25) -> ("Karte out"=w8:T1)  [unwired: 10 in]
  "Karte" <- w8
  n32 = Build Path(base path=w1, name or relative path=w12) -> (appended path=w11:path)
  n33 = Build Path(base path=w1, name or relative path=w7) -> (appended path=w5:path)
  n34 = Flatten To XML(anything=w8) -> (xml string=w16:string)
  n35 = call-poly <vilib>:"Write to XML File.vi"("XML Input"=w16, "XML File Path"=w11) -> ("error out"=w4:errorcluster)  [unwired: 7 in, 2 out]
  n36 = Write to Binary File(file (use dialog)=w5, data=w8) -> (error out=w3:errorcluster)  [unwired: 4 in, 2 out]
  n37 = Merge Errors(w4, w3) -> (→"error out":errorcluster)
